vi "VITemplate-Create Events.vi"(0 "Display State In":T2, 9 "Container State":T3, 11 "error in (no error)":errorcluster) -> (4 "Display State Out":T2, 8 "Events":T1, 15 "error out":errorcluster)   [LabVIEW 2020]
uses:
  VITemplate-Event Type.ctl
  Signal Synthesis VIs/4th Generation/Controls/SignalManager/SignalManager.xctl
  VITemplate-Event Data.ctl
  <vilib>/_xctls/Container State.ctl
  <vilib>/_xctls/XControlSupport.lvlib
  C:/Users/Ken/Desktop/XControl/State.vi
  Controls/KTable/Event Type.ctl
  Controls/KTable/KTable.xctl
  Controls/KTable/Event Data.ctl
  VITemplate-Events.ctl
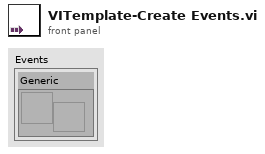
[diagram p1: front panel]
types:
  T1 = typedef "VITemplate-Events.ctl" = cluster{"Generic":refnum<user-event>}
  T2 = typedef "XControl.xctl/State.vi" = cluster{"Numeric":dbl}
  T3 = typedef "XControlSupport.lvlib/Container State.ctl" = cluster{"Indicator?":bool, "Run Mode?":bool, " Refnum":refnum<vi>}
  T4 = typedef "VITemplate-Event Data.ctl" = cluster{"Type":T5, "Data":variant}
  T5 = typedef "VITemplate-Event Type.ctl" = enum16{"None", "Selection", "Edit", "Insert", "Delete", "Up", "Down"}
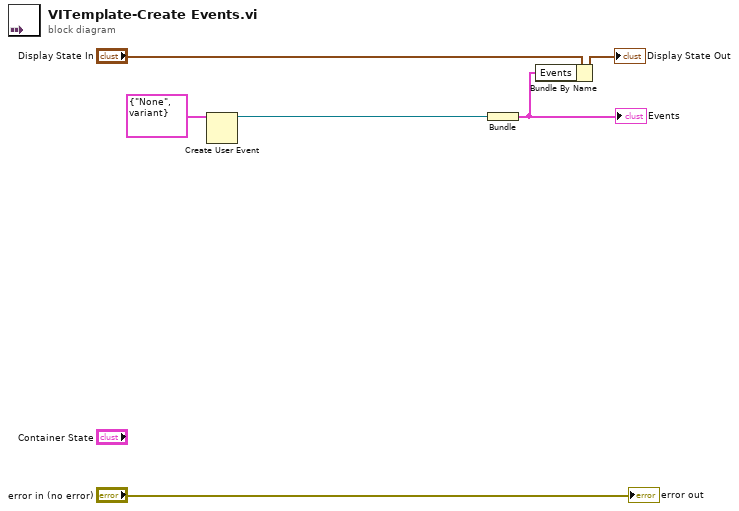
[diagram p0: block diagram]
diagram:
  n1 = Create User Event(user event datatype=T4 {"Type"=enum."None", "Data"=variant} ("Event Data")) -> (user event=w2:refnum<user-event>)  [unwired: 1 in, 1 out]
  n2 = Bundle("Event Data"=w2) -> (w1:cluster{"Event Data":refnum<user-event>})  [unwired: 1 in]
  "Events" <- w1
  n3 = Bundle By Name(cluster="Display State In", "Events"=w1) -> (→"Display State Out":T2)
  "error out" <- "error in (no error)"
